vi "XY Graph (SubVI).vi"(1 "Y":dbl, 2 "X":dbl) -> (0 "XY Graph":cluster{"array":dbl[], "array":dbl[]}(graph))   [LabVIEW 2012]
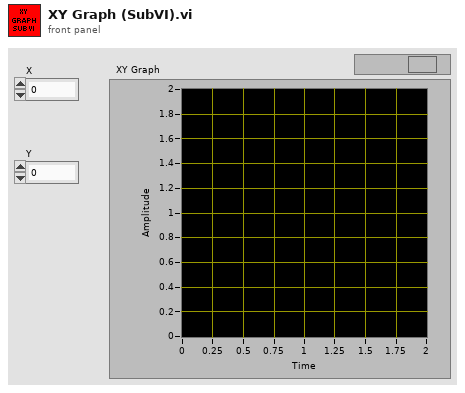
[diagram p1: front panel]
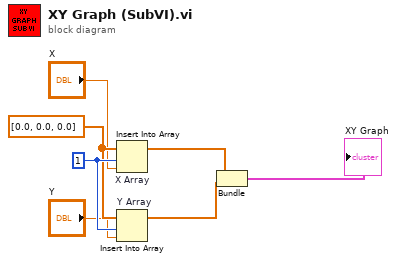
[diagram p0: block diagram]
diagram:
  w6 = dbl[] [0.0, 0.0, 0.0] ("array")
  w7 = 1 ("index")
  n1 = Insert Into Array "X Array"(array=w6, index=w7, new element="X") -> (w3:dbl[])
  n2 = Insert Into Array "Y Array"(array=w6, index=w7, new element="Y") -> (w2:dbl[])
  n3 = Bundle("array"=w3, "array"=w2) -> (→"XY Graph":cluster{"array":dbl[], "array":dbl[]})  [unwired: 1 in]
